vi "进度条.vi"(0 "error out":errorcluster, 1 "Error Out":errorcluster caption="Error in") -> ()   [LabVIEW 2012]
uses:
  <vilib>/addons/WireFlow/_WF_ProgressBar.llb/MessageTextType.ctl
  <vilib>/addons/WireFlow/_WF_ProgressBar.llb/ProgressBar_WireFlow.lvclass
panel:
  in  "delay (0 ms)":i32=1000
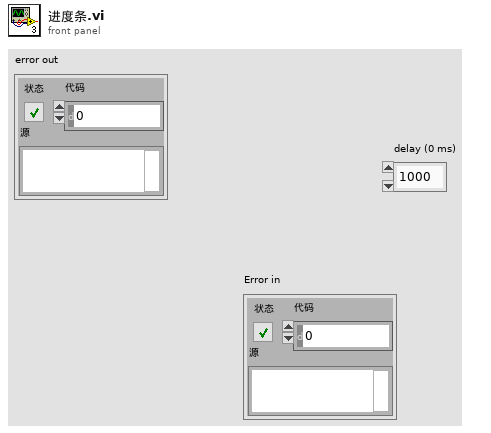
[diagram p1: front panel]
types:
  T1 = typedef "ProgressBar_WireFlow.lvclass/MessageTextType.ctl" = enum16{"Title", "General", "Current item"}
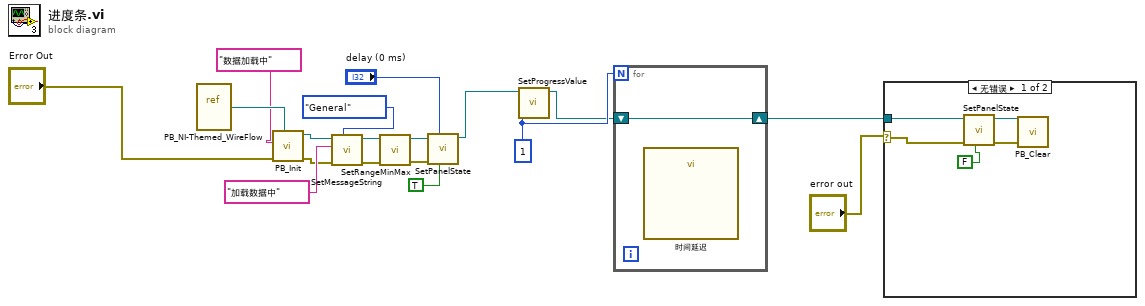
[diagram p0: block diagram]
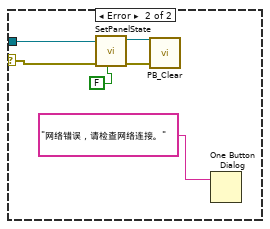
[diagram p2: hidden frame]
diagram:
  w3 = 1
  n1 = vi-ref "PB_NI-Themed_WireFlow.vi"() -> (w18:refnum<vi>)
  n2 = call <vilib>:"PB_Init.vi"("Progress VI"=w18, "error in (no error)"="Error Out", "title (\"Progress\")"="数据加载中") -> ("error out"=w11:errorcluster, "WF-ProgressBar out"=w16:refnum<class "ProgressBar_WireFlow.lvclass">)  [unwired: 7 in]
  n3 = call-dynamic "SetMessageString.vi"("message field"=MessageTextType."General", "error in (no error)"=w11, "Message"="加载数据中", "WF-ProgressBar in"=w16) -> ("error out"=w12:errorcluster, "WF-ProgressBar out"=w13:refnum<class "ProgressBar_WireFlow.lvclass">)  [unwired: 6 in]
  n4 = call-dynamic "SetRangeMinMax.vi"("error in (no error)"=w12, "WF-ProgressBar in"=w13) -> ("error out"=w9:errorcluster, "WF-ProgressBar out"=w10:refnum<class "ProgressBar_WireFlow.lvclass">)  [unwired: 8 in]
  n5 = call-dynamic "SetPanelState.vi"("State (T = Open)"=TRUE, "delay (0 ms)"="delay (0 ms)", "error in (no error)"=w9, "WF-ProgressBar in"=w10) -> ("WF-ProgressBar out"=w6:refnum<class "ProgressBar_WireFlow.lvclass">)  [unwired: 6 in, 1 out]
  n6 = call-dynamic "SetProgressValue.vi"("Value"=w3, "WF-ProgressBar in"=w6) -> ("WF-ProgressBar out"=w1:refnum<class "ProgressBar_WireFlow.lvclass">)  [unwired: 7 in, 2 out]
  n7 = for {
    N: w3 -> [_]
    shift-right: [w19] -> w2
    shift-left: w1 -> [w19]
    n8 = call "时间延迟"() -> ()  [unwired: 11 in, 1 out]
  }
  n9 = case shown="无错误" "error out" {
    selector: "error out" -> [w20 w26]
    tunnel: w2 -> [w21 w27]
    frame No Error {
      n10 = call-dynamic "SetPanelState.vi"("State (T = Open)"=FALSE, "error in (no error)"=w20, "WF-ProgressBar in"=w21) -> ("error out"=w22:errorcluster, "WF-ProgressBar out"=w23:refnum<class "ProgressBar_WireFlow.lvclass">)  [unwired: 7 in]
      n11 = call-dynamic "PB_Clear.vi"("error in (no error)"=w22, "WF-ProgressBar in"=w23) -> ()  [unwired: 8 in, 2 out]
    }
    frame Error {
      n12 = call-dynamic "SetPanelState.vi"("State (T = Open)"=FALSE, "error in (no error)"=w26, "WF-ProgressBar in"=w27) -> ("error out"=w28:errorcluster, "WF-ProgressBar out"=w29:refnum<class "ProgressBar_WireFlow.lvclass">)  [unwired: 7 in]
      n13 = call-dynamic "PB_Clear.vi"("error in (no error)"=w28, "WF-ProgressBar in"=w29) -> ()  [unwired: 8 in, 2 out]
      n14 = One Button Dialog(message="网络错误，请检查网络连接。") -> ()  [unwired: 1 in, 1 out]
    }
  }
